vi "OpenCollector.vi"(8 "error in (no error)":errorcluster, 9 "Ram?":bool, 10 "path to db monitoring":path, 11 "DataCollector in":refnum<class "DataCollector.lvclass">) -> (0 "error out":errorcluster, 2 "Rows = 0?":bool, 3 "DataCollector out":refnum<class "DataCollector.lvclass">)   [LabVIEW 2017, in "DataCollector.lvclass"]
uses:
  DataCollector.lvclass
  <vilib>/drjdpowell/SQLite Library/SQL Connection/Connection.lvclass
  <vilib>/drjdpowell/SQLite Library/SQL Connection/Open (path).vi
  <vilib>/drjdpowell/SQLite Library/SQL Connection/Open (string).vi
  <vilib>/drjdpowell/SQLite Library/SQLite.lvlib
  <vilib>/drjdpowell/SQLite Library/SQL Connection/Execute SQL.vi
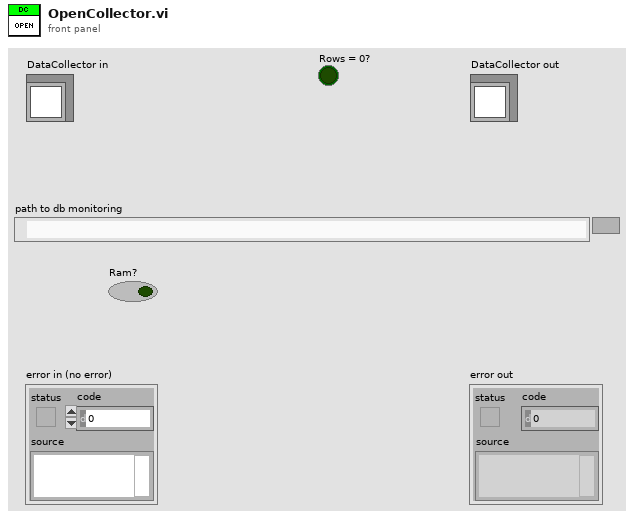
[diagram p1: front panel]
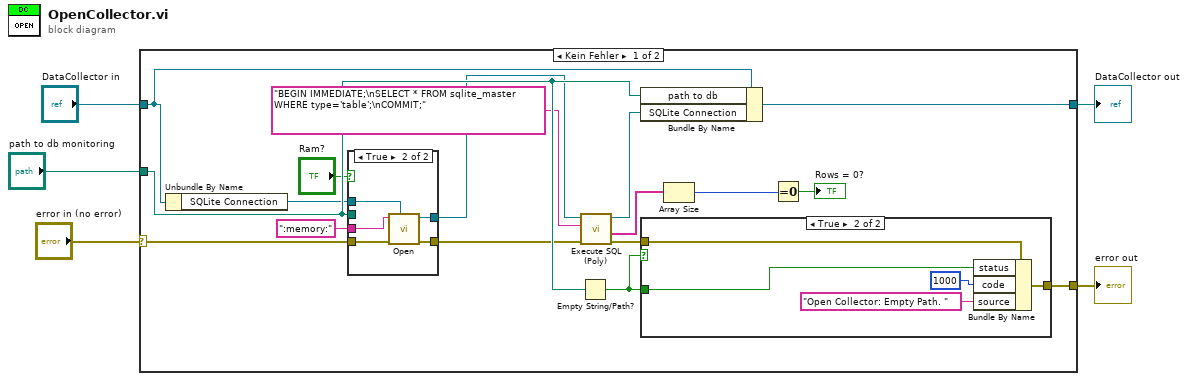
[diagram p0: block diagram]
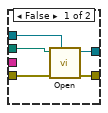
[diagram p2: hidden frame]
diagram:
  n1 = case shown="Kein Fehler" "error in (no error)" {
    selector: "error in (no error)" -> [w22 w39]
    tunnel: [w19 w39] -> w4
    tunnel: [w21 w40] -> w2
    tunnel: "DataCollector in" -> [w20 w40]
    tunnel: "path to db monitoring" -> [w17 _]
    frame No Error {
      n2 = Unbundle By Name(w20) -> ("SQLite Connection"=w14:refnum<class "Connection.lvclass">)
      n3 = case shown="True" "Ram?" {
        tunnel: w22 -> [w27 w32]
        tunnel: w14 -> [w26 w29]
        tunnel: [w25 w30] -> w12
        tunnel: [w24 w31] -> w10
        tunnel: w17 -> [w23 _]
        tunnel: ":memory:" -> [_ w28]
        frame False {
          n4 = call-poly <vilib>:"Open.vi"("SQLite Connection type"=w26, "error in (no error)"=w27, "db file"=w23) -> ("error out"=w24:errorcluster, "SQLite Connection"=w25:refnum<class "Connection.lvclass">)  [unwired: 7 in]
        }
        frame True {
          n5 = call-poly <vilib>:"Open.vi"("SQLite Connection type"=w29, "error in (no error)"=w32, "db file"=w28) -> ("error out"=w31:errorcluster, "SQLite Connection"=w30:refnum<class "Connection.lvclass">)  [unwired: 7 in]
        }
      }
      n6 = Empty String/Path?(string/path=w17) -> (empty?=w18:bool)
      n7 = call-poly <vilib>:"Execute SQL (Poly).vi"("error in (no error)"=w10, "SQL"="BEGIN IMMEDIATE;\nSELECT * FROM sqlite_master WHERE type='table';\nCOMMIT;" ("String"), "SQLite Connection in"=w12) -> ("error out"=w9:errorcluster, "Column Names"=w8:string[], "SQLite Connection"=w11:refnum<class "Connection.lvclass">)  [unwired: 5 in, 1 out]
      n8 = Bundle By Name(cluster=w20, "path to db"=w17, "SQLite Connection"=w11) -> (w21:refnum<class "DataCollector.lvclass">)
      n9 = case shown="True" w18 {
        tunnel: w9 -> [w33 w36]
        tunnel: [w33 w35] -> w19
        tunnel: w18 -> [_ w34]
        frame False {
        }
        frame True {
          n10 = Bundle By Name(cluster=w36, "status"=w34, "code"=1000, "source"="Open Collector: Empty Path. ") -> (w35:errorcluster)
        }
      }
      n11 = Array Size(array=w8) -> (size(s)=w7:i32)
      n12 = Equal To 0?(x=w7) -> (x = 0?=→"Rows = 0?":bool)
    }
    frame Error {
    }
  }
  "error out" <- w4
  "DataCollector out" <- w2
